vi "Value Allready existe.vi"(8 "error in (no error)":errorcluster caption="entrée d'erreur (pas d'erreur)", 10 "Parameter":T1, 11 "Database Altyor en entrée":refnum<class "Database Altyor Packaging.lvclass">) -> (0 "error out":errorcluster caption="sortie d'erreur", 1 "Data_Read":variant[][](array[variant]), 2 "All ready Existe":bool=TRUE, 3 "Database Altyor en sortie":refnum<class "Database Altyor Packaging.lvclass">)   [LabVIEW 2020, in "Library Instrument & Equipement.lvlib" / "Library Database.lvlib" / "Database Altyor Packaging.lvclass"]
uses:
  Database Altyor Packaging.lvclass
  C:/Users/ngarcin/OneDrive - Altyor/Standard TB/Class/Database/Database drivers/Database Drivers.lvclass
  Database Altyor Packaging.lvclass/Database Altyor Packaging.ctl
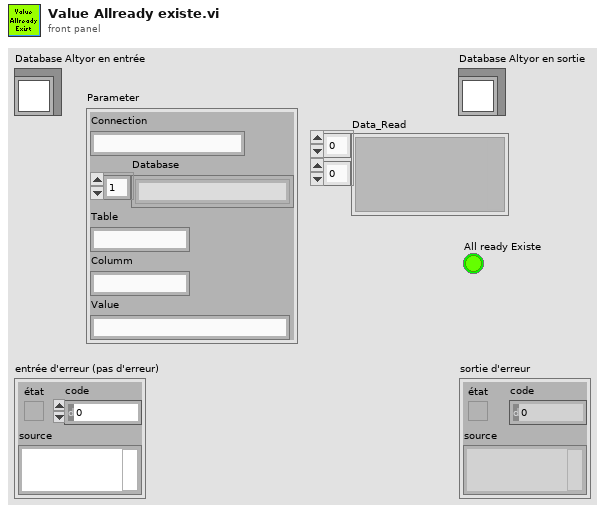
[diagram p1: front panel]
types:
  T1 = cluster{"Connection":string, "Database":string[], "Table":string, "Columm":string, "Value":string}
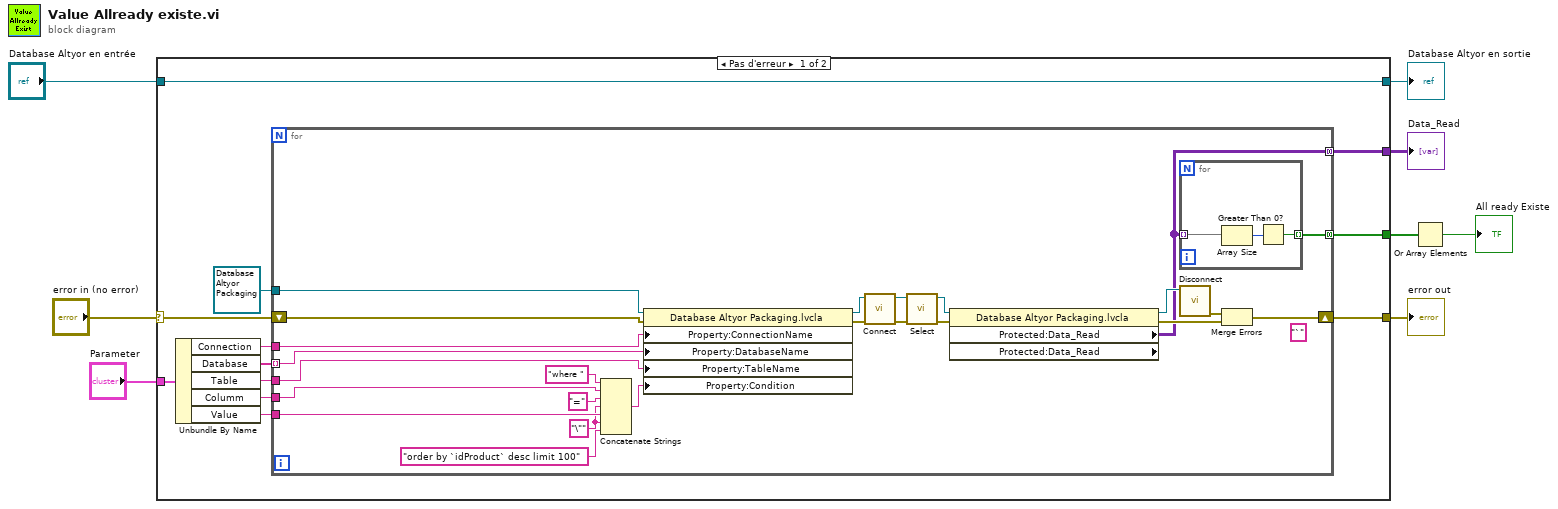
[diagram p0: block diagram]
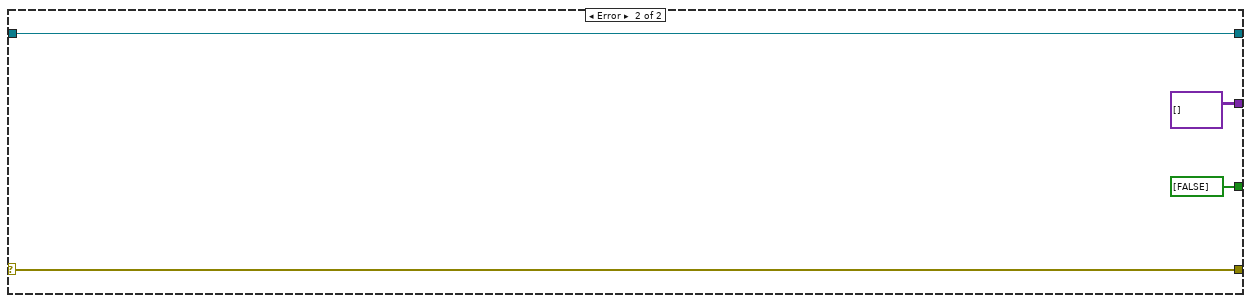
[diagram p2: hidden frame]
diagram:
  n1 = case shown="Pas d'erreur" "error in (no error)" {
    selector: "error in (no error)" -> [w13 w51]
    tunnel: [w12 w51] -> w7
    tunnel: [w20 w50] -> w5
    tunnel: "Database Altyor en entrée" -> [w20 w50]
    tunnel: "Parameter" -> [w19 _]
    tunnel: [w11 bool[] [FALSE]] -> w3
    tunnel: [w9 variant[][] [] ("Protected:Data_Read")] -> w1
    frame No Error {
      n2 = Unbundle By Name(w19) -> ("Connection"=w17:string, "Database"=w16:string[], "Table"=w15:string, "Columm"=w18:string, "Value"=w10:string)
      n3 = for {
        tunnel: w18 -> [w23]
        tunnel: w17 -> [w42]
        tunnel: w16 -> [w41] mode=indexing
        tunnel: w15 -> [w25]
        tunnel: refnum<class "Database Altyor Packaging.lvclass"> refnum ("Library Instrument & Equipement.lvlib:Library Database.lvlib:Database Altyor.lvclass") -> [w40]
        shift-right: [w31] -> w12
        shift-left: w13 -> [w39]
        tunnel: [w29] -> w11 mode=concatenating
        tunnel: w10 -> [w27]
        tunnel: [w21] -> w9 mode=concatenating
        (unwired) "`" ("chaîne")
        w26 = "\"" ("chaîne")
        n4 = Concatenate Strings("where " ("Condition"), w23, "=" ("Condition"), w26, w27, w26, "order by `idProduct` desc limit 100" ("chaîne")) -> (w28:string)
        n5 = property class="Database Altyor Packaging.lvcla"(reference=w40, error in=w39, "Property:ConnectionName"=w42, "Property:DatabaseName"=w41, "Property:TableName"=w25, "Property:Condition"=w28) -> (reference out=w36:refnum<class "Database Altyor Packaging.lvclass">, error out=w37:errorcluster)
        n6 = call-dynamic "Connect.vi"("error in (no error)"=w37, "Database Altyor en entrée"=w36) -> ("error out"=w38:errorcluster, "Database Altyor en sortie"=w35:refnum<class "Database Altyor Packaging.lvclass">)  [unwired: 8 in]
        n7 = call-dynamic "Select.vi"("error in (no error)"=w38, "Database Drivers en entrée"=w35) -> ("error out"=w44:errorcluster, "Database Drivers en sortie"=w43:refnum<class "Database Altyor Packaging.lvclass">)  [unwired: 8 in]
        n8 = property class="Database Altyor Packaging.lvcla" props=["Protected:Data_Read", "Protected:Data_Read"](reference=w43, error in=w44) -> (reference out=w34:refnum<class "Database Altyor Packaging.lvclass">, error out=w33:errorcluster, "Protected:Data_Read"=w21:variant[][])  [unwired: 1 out]
        n9 = for {
          tunnel: w21 -> [w47] mode=indexing
          tunnel: [w45] -> w29 mode=indexing
          n10 = Array Size(array=w47) -> (size(s)=w46:i32)
          n11 = Greater Than 0?(x=w46) -> (x > 0?=w45:bool)
        }
        n12 = call-dynamic "Disconnect.vi"("Database Altyor en entrée"=w34) -> ("error out"=w32:errorcluster)  [unwired: 9 in, 1 out]
        n13 = Merge Errors(w32, w33) -> (w31:errorcluster)
      }
    }
    frame Error {
    }
  }
  "error out" <- w7
  "Database Altyor en sortie" <- w5
  "Data_Read" <- w1
  n14 = Or Array Elements(Boolean array=w3) -> (logical OR=→"All ready Existe":bool)
